vi "Package Measurement Plugin.vi"() -> ()   [LabVIEW 2021]
uses:
  _Measurement Plugin Packager/Packager Helpers/Queue Driver/controls/Queue Operations.ctl
  <vilib>/Utility/miscctls.llb/LVRowAndColumnTypeDef.ctl
  _Measurement Plugin Packager/Packager Helpers/controls/Config File Operations.ctl
  _Measurement Plugin Packager/Packager Helpers/controls/Data Holder.ctl
  <vilib>/Utility/miscctls.llb/LVPoint32TypeDef.ctl
  _Measurement Plugin Packager/Packager Helpers/controls/Build Spec Details.ctl
  <vilib>/AppBuilder/AB_API_Simple/Get Build Specification Version (path).vi
  _Measurement Plugin Packager/Packager Helpers/Queue Driver/Queue Driver.lvlib
  _Measurement Plugin Packager/Packager Helpers/Packager Helpers.lvlib
  _Measurement Plugin Packager/Packager Helpers/Dictionary/Dictionary.lvlib
  <vilib>/AppBuilder/AB_API_Simple/NI_App_Builder_API.lvlib
panel:
  out "error out":errorcluster
  out "Tab Control":T1(tab)
  in  "Open Directory":bool
  in  "Feed Path":path
  out "Warning":bool=TRUE caption="Existing LabVIEW Project Path should be selected"
  in  "Next to select":bool
  in  "Project":path caption="LabVIEW Project Path"
  in  "Feed":T2(radio)
  in  "Back 1":bool
  in  "Populate Package":bool
  in  "Select All":bool
  out "Measurement List":i32(listbox)=-1 caption="Select the Measurements to build the package"
  out "Selection warning":string="Selected Project doesn't have EXE build spec"
  out "Maintainer Warning":string
  in  "Settings Page":enum32{"Page 1", "Page 2"}(tab)
  in  "Maintainer Email ID":string="sabthagiri@ni.com"
  in  "Architecture":string(combo)="1"
  in  "Maintainer":string="NI"
  in  "Back 2":bool
  in  "Start Build":bool
  in  "Package List":i32[](listbox) caption="Edit the Package Name and Version"
  in  "Settings":bool
  in  "Progres Bar":i32(slide)=9 caption="Creating Distribution..." scale=0.0..100.0
  in  "Start Next":bool
  in  "Build Status":i32(listbox)=-1
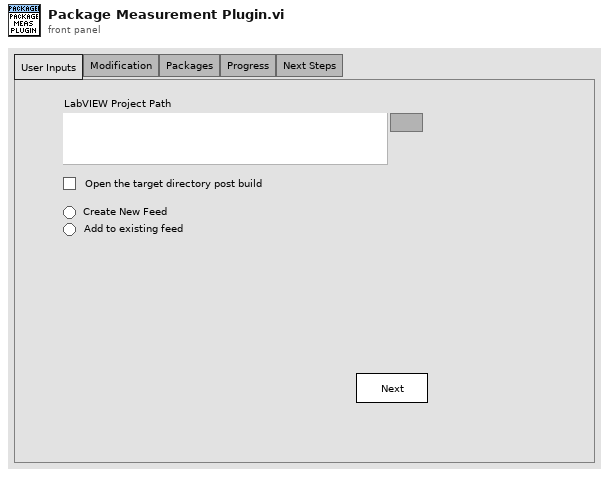
[diagram p1: front panel]
types:
  T1 = enum32{"User Inputs", "Modification", "Packages", "Progress", "Next Steps"}
  T2 = enum32{"No Selection", "CreateFeed", "AddtoFeed"}
  T3 = typedef "LVRowAndColumnTypeDef.ctl" = cluster{"Row":i32, "Column":i32}
  T4 = typedef "Queue Driver.lvlib/Queue Operations.ctl" = enum16{"Create Q", "Enqueue", "Enqueue N", "Dequeue", "Flush", "Release"}
  T5 = enum8{"Enabled", "Disabled", "Disabled and Grayed Out"}
  T6 = typedef "Packager Helpers.lvlib/Config File Operations.ctl" = enum16{"Read", "Write"}
  T7 = typedef "Packager Helpers.lvlib/Data Holder.ctl" = cluster{"Next Clicked?":bool, "MosueDown Coords":T8, "Build Spec":T9[], "No of Meas":i32, "No. of Selected Meas":i32, "Selected Meas":T9[], "Package Details":string[][], "Packages Path":path, "Feed":enum32{"No Selection", "CreateFeed", "AddtoFeed"}, "Feed Path":path, "Valid Inputs?":bool, "Feed Old":enum32{"No Selection", "CreateFeed", "AddtoFeed"}, "Status":string[], "Open Directory?":bool}
  T8 = typedef "LVPoint32TypeDef.ctl" = cluster{"Horizontal":i32, "Vertical":i32}
  T9 = typedef "Packager Helpers.lvlib/Build Spec Details.ctl" = cluster{"EXE Name":string, "Target path":path, "Has PPL?":bool, "PPL Name":string}
  T10 = typedef "NI_App_Builder_API.lvlib/Build Specification Version.ctl" = cluster{"Major":u16, "Minor":u16, "Fix":u16, "Build":u16}
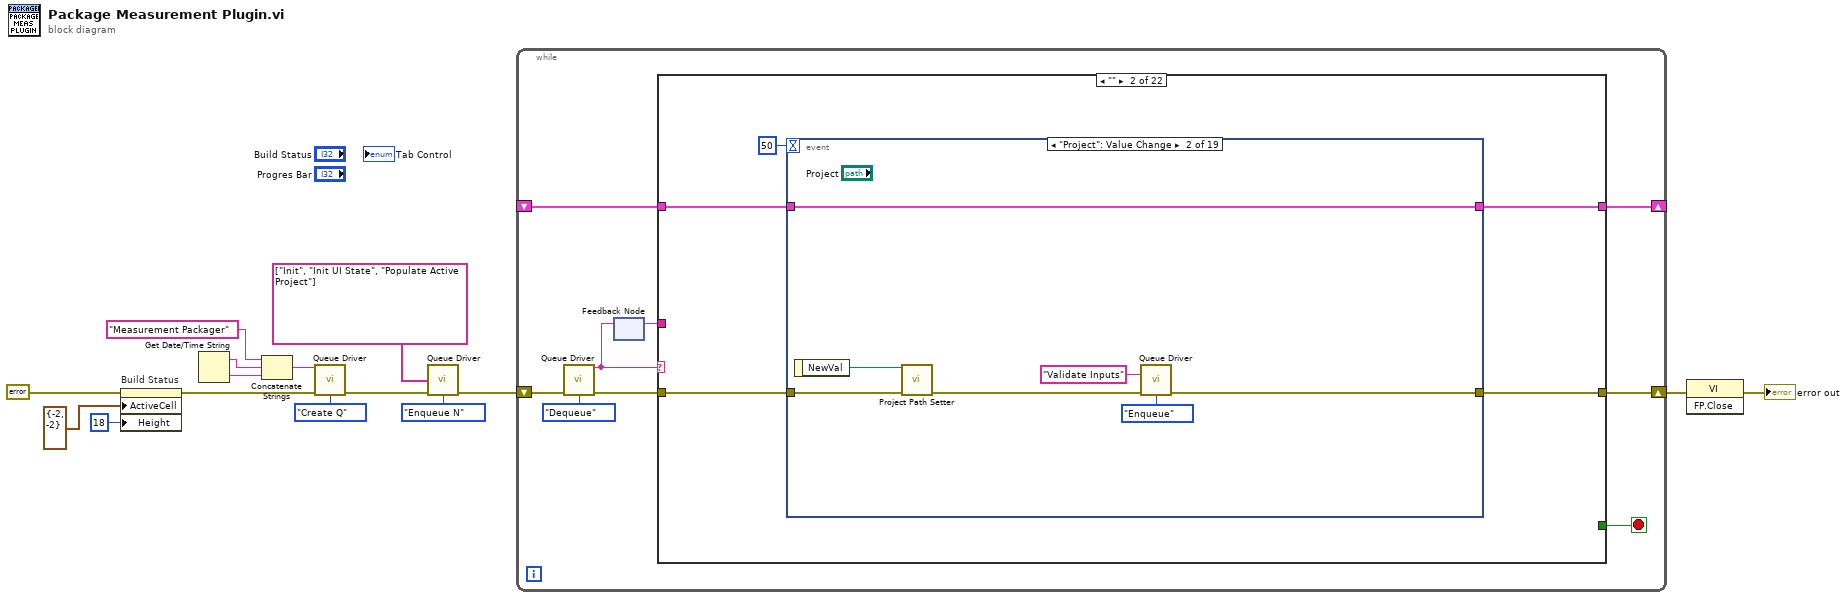
[diagram p0: block diagram]
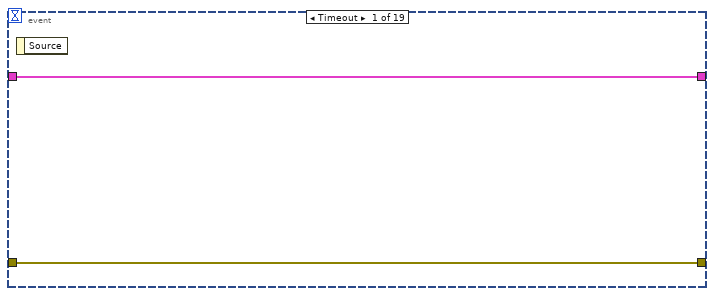
[diagram p3: hidden frame]
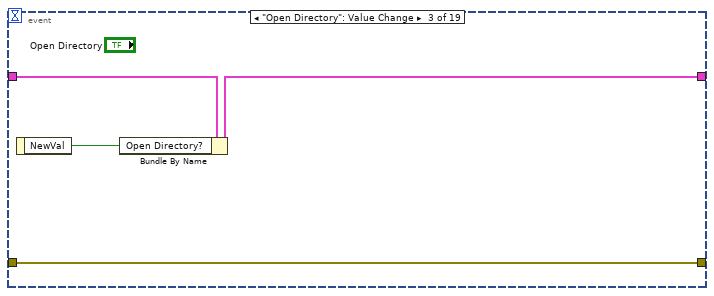
[diagram p4: hidden frame]
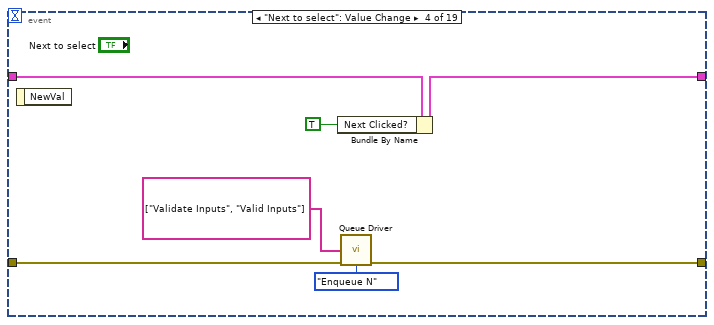
[diagram p5: hidden frame]
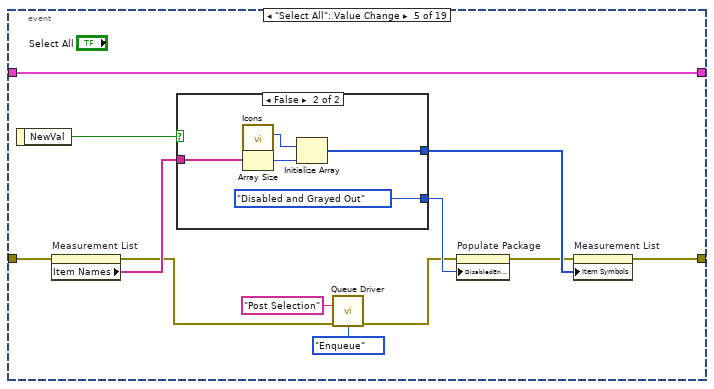
[diagram p6: hidden frame]
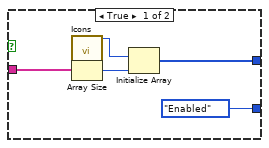
[diagram p7: hidden frame]
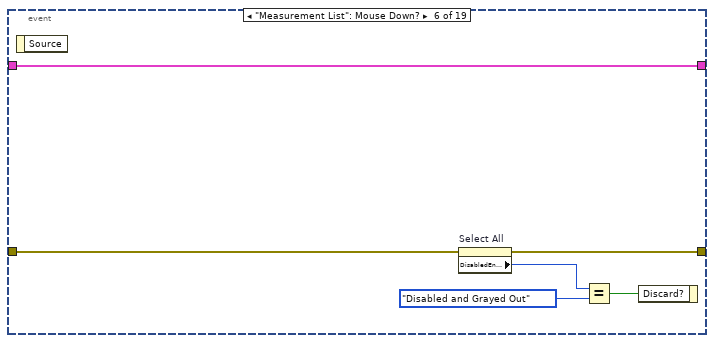
[diagram p8: hidden frame]
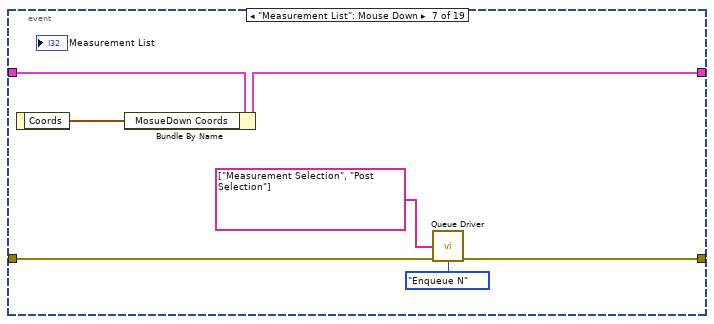
[diagram p9: hidden frame]
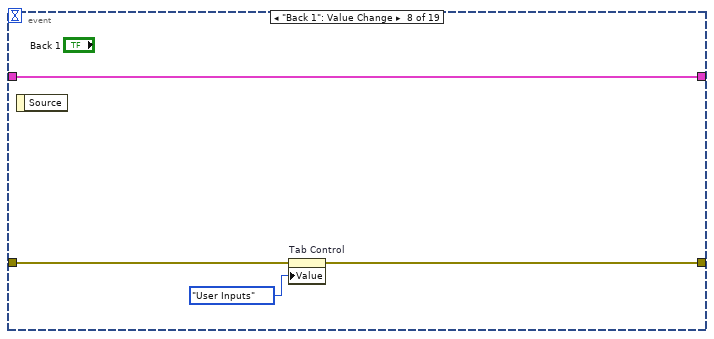
[diagram p10: hidden frame]
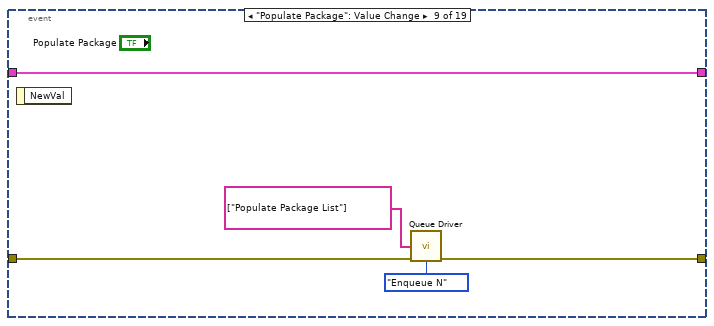
[diagram p11: hidden frame]
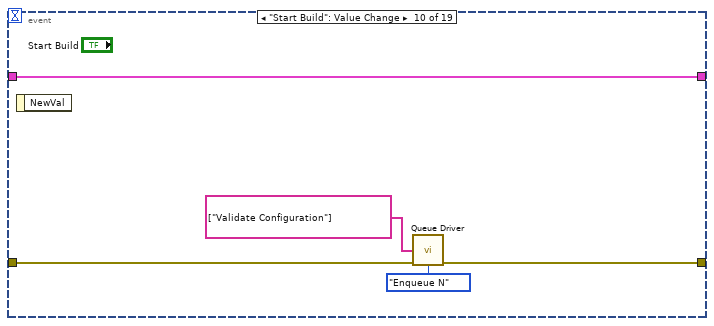
[diagram p12: hidden frame]
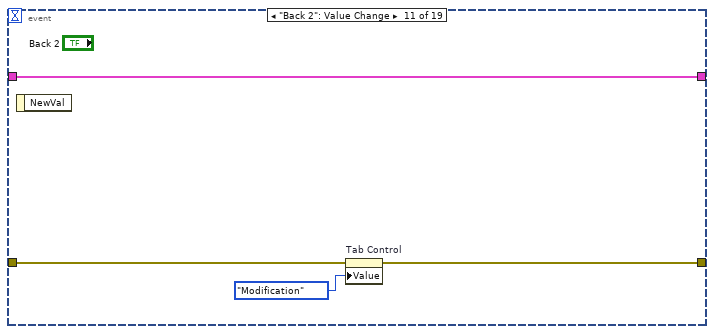
[diagram p13: hidden frame]
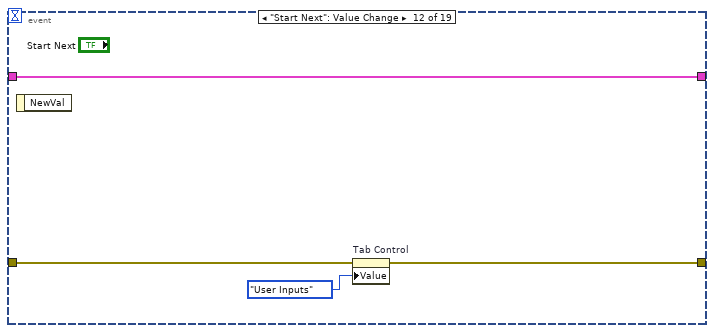
[diagram p14: hidden frame]
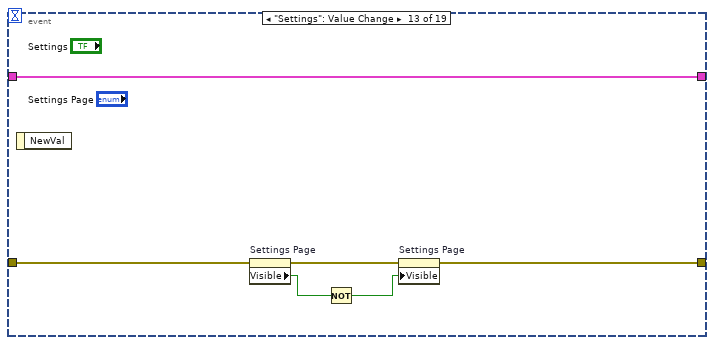
[diagram p15: hidden frame]
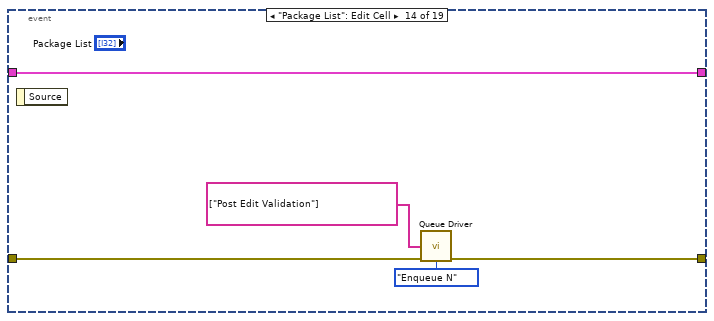
[diagram p16: hidden frame]
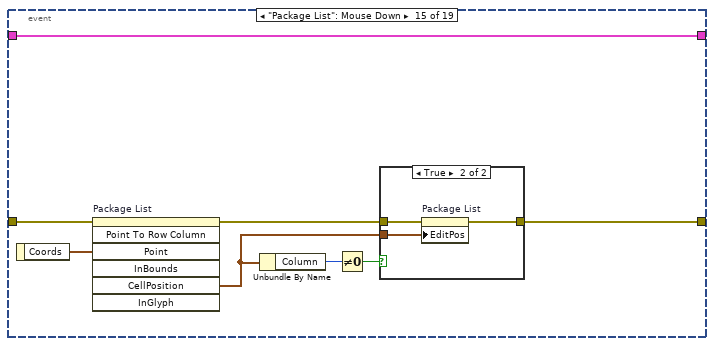
[diagram p17: hidden frame]
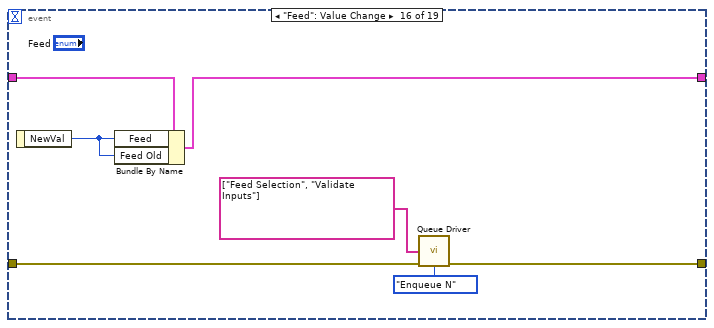
[diagram p19: hidden frame]
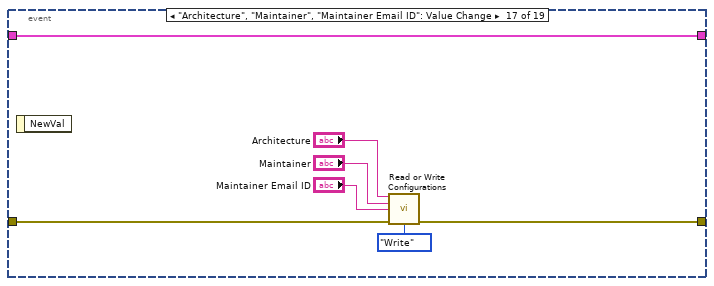
[diagram p20: hidden frame]
diagram:
  n1 = property on="Build Status" class="MCListbox (strict)"(error in=errorcluster {"status"=FALSE, "code"=0, "source"=""} ("error in (no error)"), "ActiveCell"=T3 {"Row"=-2, "Column"=-2} ("Active Cell:Active Cell"), "Height"=u32 18 ("Active Cell:Cell Size:Height")) -> (error out=w1:errorcluster)  [unwired: 1 in, 1 out]
  n2 = Get Date/Time String() -> (date string=w4:string, time string=w10:string)  [unwired: 3 in]
  n3 = Concatenate Strings("Measurement Packager" ("string"), w4, w10) -> (w9:string)
  n4 = call "Queue Driver.vi"("Name"=w9, "error in (no error)"=w1, "Queue Operations"=Queue_Operations."Create Q" ("Q Operations")) -> ("error out"=w13:errorcluster)  [unwired: 11 in, 1 out]
  n5 = call "Queue Driver.vi"("States[]"=string[] ["Init", "Init UI State", "Populate Active Project"], "error in (no error)"=w13, "Queue Operations"=Queue_Operations."Enqueue N" ("Q Operations")) -> ("error out"=w15:errorcluster)  [unwired: 11 in, 1 out]
  n6 = while {
    shift-right: [w17] -> w6
    shift-left: w15 -> [w24]
    shift-right: [w21] -> _
    shift-left: _ -> [w20]
    stop <- w18 stop-if-true
    n7 = call "Queue Driver.vi"("error in (no error)"=w24, "Queue Operations"=Queue_Operations."Dequeue" ("Q Operations")) -> ("Dequeued State"=w16:string, "error out"=w22:errorcluster)  [unwired: 12 in]
    n8 = feedback #1() -> (w19:string)  [unwired: 1 in]
    n9 = feedback-in #1(w16) -> ()
    n10 = case shown="\"\"" w16 {
      tunnel: w22 -> [w25 w31 w163 w176 w187 w190 w203 w243 w258 w273 w296 w315 w329 w336 w356 w392 w396 w410 w425 w439 w452 w457]
      tunnel: [w25 w27 w161 w167 w184 w189 w206 w242 w257 w270 w288 w316 w328 w333 w350 w391 w394 w407 w420 w437 w448 w459] -> w17
      tunnel: [w26 w30 w164 w179 w188 w191 w205 w241 w259 w275 w298 w323 w331 w342 w359 w393 w397 w403 w436 w441 w455 w460] -> w21
      tunnel: w20 -> [w26 w29 _ w179 w188 w191 w204 w241 w259 w275 w298 w324 w331 w342 w357 w393 w399 w403 w432 w441 w455 w460]
      tunnel: w19 -> [_ _ _ _ _ _ _ _ _ _ _ _ _ _ _ _ _ _ _ _ _ _]
      tunnel: [_ _ _ _ _ _ _ _ _ _ _ _ _ _ _ _ _ _ _ _ _ TRUE] -> w18
      frame Default {
      }
      frame "" {
        n11 = event shown="[1] \"Project\": Value Change" {
          selector: _ -> [_ _ _ _ _ _ _ _ _ _ _ _ _ _ _ _ _ _ _]
          dyn-events: _ -> [_ _ _ _ _ _ _ _ _ _ _ _ _ _ _ _ _ _ _]
          timeout: 50 -> [_ _ _ _ _ _ _ _ _ _ _ _ _ _ _ _ _ _ _]
          tunnel: [w32 w34 w41 w45 w52 w77 w81 w87 w93 w96 w103 w107 w111 w115 w121 w133 w139 w147 w153] -> w27
          tunnel: w31 -> [w32 w36 w41 w46 w56 w78 w80 w88 w94 w97 w104 w108 w112 w116 w120 w134 w140 w148 w154]
          tunnel: [w33 w39 w43 w49 w63 w79 w85 w90 w95 w100 w102 w106 w109 w119 w127 w137 w145 w151 w157] -> w30
          tunnel: w29 -> [w33 w39 w44 w50 w63 w79 w86 w90 w95 w100 w102 w106 w109 w119 w127 w138 w145 w152 w157]
          event Timeout {
            n12 = event-data() -> ()  [unwired: 1 in, 1 out]
          }
          event "Project": Value Change {
            n13 = event-data() -> ("NewVal"=w38:path)  [unwired: 1 in]
            n14 = call "Project Path Setter.vi"("ProjectPath In"=w38, "error in (no error)"=w36) -> ("error out"=w35:errorcluster)  [unwired: 13 in]
            n15 = call "Queue Driver.vi"("State"="Validate Inputs", "error in (no error)"=w35, "Queue Operations"=Queue_Operations."Enqueue" ("Q Operations")) -> ("error out"=w34:errorcluster)  [unwired: 11 in, 1 out]
          }
          event "Open Directory": Value Change {
            n16 = event-data() -> ("NewVal"=w42:bool)  [unwired: 1 in]
            n17 = Bundle By Name(cluster=w44, "Open Directory?"=w42) -> (w43:T7)
          }
          event "Next to select": Value Change {
            n18 = event-data() -> ()  [unwired: 1 in, 1 out]
            n19 = Bundle By Name(cluster=w50, "Next Clicked?"=TRUE) -> (w49:T7)
            n20 = call "Queue Driver.vi"("States[]"=string[] ["Validate Inputs", "Valid Inputs"], "error in (no error)"=w46, "Queue Operations"=Queue_Operations."Enqueue N" ("Q Operations")) -> ("error out"=w45:errorcluster)  [unwired: 11 in, 1 out]
          }
          event "Select All": Value Change {
            n21 = event-data() -> ("NewVal"=w58:bool)  [unwired: 1 in]
            n22 = property on="Measurement List" class="LstBox (strict)"(error in=w56) -> (error out=w55:errorcluster, "Item Names"=w62:string[])  [unwired: 1 in, 1 out]
            n23 = case shown="False" w58 {
              tunnel: w62 -> [w67 w72]
              tunnel: [w66 w71] -> w61
              tunnel: [T5."Enabled" ("Disabled") T5."Disabled and Grayed Out" ("Disabled")] -> w60
              frame True {
                n24 = call "Icons.vi"() -> ("Selected"=w64:i32)  [unwired: 14 in, 1 out]
                n25 = Array Size(array=w67) -> (size(s)=w68:i32)
                n26 = Initialize Array(w64, w68) -> (w66:i32[])
              }
              frame False {
                n27 = call "Icons.vi"() -> ("Non Selected"=w70:i32)  [unwired: 14 in, 1 out]
                n28 = Array Size(array=w72) -> (size(s)=w73:i32)
                n29 = Initialize Array(w70, w73) -> (w71:i32[])
              }
            }
            n30 = call "Queue Driver.vi"("State"="Post Selection", "error in (no error)"=w55, "Queue Operations"=Queue_Operations."Enqueue" ("Q Operations")) -> ("error out"=w54:errorcluster)  [unwired: 11 in, 1 out]
            n31 = property on="Populate Package" class="Bool"(error in=w54, "DisabledEnum"=w60) -> (error out=w53:errorcluster)  [unwired: 1 in, 1 out]
            n32 = property on="Measurement List" class="LstBox (strict)"(error in=w53, "Item Symbols"=w61) -> (error out=w52:errorcluster)  [unwired: 1 in, 1 out]
          }
          event "Measurement List": Mouse Down? {
            n33 = event-data() -> ()  [unwired: 1 in, 1 out]
            n34 = property on="Select All" class="Bool (strict)"(error in=w78) -> (error out=w77:errorcluster, "DisabledEnum"=w76:T5)  [unwired: 1 in, 1 out]
            n35 = Equal?(x=w76, y=T5."Disabled and Grayed Out") -> (x = y?=w74:bool)
            n36 = event-data("Discard?"=w74) -> ()  [unwired: 1 in, 1 out]
          }
          event "Measurement List": Mouse Down {
            n37 = event-data() -> ("Coords"=w83:T8)  [unwired: 1 in]
            n38 = Bundle By Name(cluster=w86, "MosueDown Coords"=w83) -> (w85:T7)
            n39 = call "Queue Driver.vi"("States[]"=string[] ["Measurement Selection", "Post Selection"], "error in (no error)"=w80, "Queue Operations"=Queue_Operations."Enqueue N" ("Q Operations")) -> ("error out"=w81:errorcluster)  [unwired: 11 in, 1 out]
          }
          event "Back 1": Value Change {
            n40 = event-data() -> ()  [unwired: 1 in, 1 out]
            n41 = property on="Tab Control" class="TabCtl (strict)"(error in=w88, "Value"=T1."User Inputs" ("Tab Control")) -> (error out=w87:errorcluster)  [unwired: 1 in, 1 out]
          }
          event "Populate Package": Value Change {
            n42 = event-data() -> ()  [unwired: 1 in, 1 out]
            n43 = call "Queue Driver.vi"("States[]"=string[] ["Populate Package List"], "error in (no error)"=w94, "Queue Operations"=Queue_Operations."Enqueue N" ("Q Operations")) -> ("error out"=w93:errorcluster)  [unwired: 11 in, 1 out]
          }
          event "Start Build": Value Change {
            n44 = event-data() -> ()  [unwired: 1 in, 1 out]
            n45 = call "Queue Driver.vi"("States[]"=string[] ["Validate Configuration"], "error in (no error)"=w97, "Queue Operations"=Queue_Operations."Enqueue N" ("Q Operations")) -> ("error out"=w96:errorcluster)  [unwired: 11 in, 1 out]
          }
          event "Back 2": Value Change {
            n46 = event-data() -> ()  [unwired: 1 in, 1 out]
            n47 = property on="Tab Control" class="TabCtl (strict)"(error in=w104, "Value"=T1."Modification" ("Tab Control")) -> (error out=w103:errorcluster)  [unwired: 1 in, 1 out]
          }
          event "Start Next": Value Change {
            n48 = event-data() -> ()  [unwired: 1 in, 1 out]
            n49 = property on="Tab Control" class="TabCtl (strict)"(error in=w108, "Value"=T1."User Inputs" ("Tab Control")) -> (error out=w107:errorcluster)  [unwired: 1 in, 1 out]
          }
          event "Settings": Value Change {
            n50 = event-data() -> ()  [unwired: 1 in, 1 out]
            n51 = property on="Settings Page" class="TabCtl (strict)"(error in=w112) -> (error out=w110:errorcluster, "Visible"=w114:bool)  [unwired: 1 in, 1 out]
            n52 = Not(x=w114) -> (.not. x?=w113:bool)
            n53 = property on="Settings Page" class="TabCtl (strict)"(error in=w110, "Visible"=w113) -> (error out=w111:errorcluster)  [unwired: 1 in, 1 out]
          }
          event "Package List": Edit Cell {
            n54 = event-data() -> ()  [unwired: 1 in, 1 out]
            n55 = call "Queue Driver.vi"("States[]"=string[] ["Post Edit Validation"], "error in (no error)"=w116, "Queue Operations"=Queue_Operations."Enqueue N" ("Q Operations")) -> ("error out"=w115:errorcluster)  [unwired: 11 in, 1 out]
          }
          event "Package List": Mouse Down {
            n56 = event-data() -> ("Coords"=w126:T8)  [unwired: 1 in]
            n57 = invoke on="Package List" class="MCListbox (strict)" method="Point To Row Column"(error in=w120, "Point"=w126) -> (error out=w122:errorcluster, "CellPosition"=w123:T3)  [unwired: 5 in, 5 out]
            n58 = Unbundle By Name(w123) -> ("Column"=w125:i32)
            n59 = Not Equal To 0?(x=w125) -> (x != 0?=w124:bool)
            n60 = case shown="True" w124 {
              tunnel: w123 -> [_ w131]
              tunnel: w122 -> [w128 w130]
              tunnel: [w128 w129] -> w121
              frame False {
              }
              frame True {
                n61 = property on="Package List" class="MCListbox (strict)"(error in=w130, "EditPos"=w131) -> (error out=w129:errorcluster)  [unwired: 1 in, 1 out]
              }
            }
          }
          event "Feed": Value Change {
            n62 = event-data() -> ("NewVal"=w132:T2)  [unwired: 1 in]
            n63 = Bundle By Name(cluster=w138, "Feed"=w132, "Feed Old"=w132) -> (w137:T7)
            n64 = call "Queue Driver.vi"("States[]"=string[] ["Feed Selection", "Validate Inputs"], "error in (no error)"=w134, "Queue Operations"=Queue_Operations."Enqueue N" ("Q Operations")) -> ("error out"=w133:errorcluster)  [unwired: 11 in, 1 out]
          }
          event "Architecture", "Maintainer", "Maintainer Email ID": Value Change {
            n65 = event-data() -> ()  [unwired: 1 in, 1 out]
            n66 = call "Read or Write Configurations.vi"("Architecture"="Architecture", "Maintainer"="Maintainer", "Email"="Maintainer Email ID", "error in (no error)"=w140, "Operation"=Config_File_Operations."Write") -> ("error out"=w139:errorcluster)  [unwired: 7 in, 3 out]
          }
          event "Feed Path": Value Change {
            n67 = event-data() -> ("NewVal"=w149:path)  [unwired: 1 in]
            n68 = Bundle By Name(cluster=w152, "Feed Path"=w149) -> (w151:T7)
            n69 = call "Queue Driver.vi"("States[]"=string[] ["Validate Inputs"], "error in (no error)"=w148, "Queue Operations"=Queue_Operations."Enqueue N" ("Q Operations")) -> ("error out"=w147:errorcluster)  [unwired: 11 in, 1 out]
          }
          event Panel Close? {
            n70 = event-data() -> ()  [unwired: 1 in, 4 out]
            n71 = call "Queue Driver.vi"("State"="Exit", "error in (no error)"=w154, "Queue Operations"=Queue_Operations."Enqueue" ("Q Operations")) -> ("error out"=w153:errorcluster)  [unwired: 11 in, 1 out]
            n72 = event-data("Discard?"=TRUE) -> ()  [unwired: 1 in, 1 out]
          }
        }
      }
      frame "Init" {
        w160 = TRUE ("Open Directory?")
        w159 = T2."No Selection" ("Feed")
        n73 = invoke class="VI" method="Default Vals.Reinit All"(error in=w163) -> (error out=w162:errorcluster)  [unwired: 2 in, 2 out]
        n74 = property on="Open Directory" class="Bool (strict)"(error in=w162, "Value"=w160) -> (error out=w161:errorcluster)  [unwired: 1 in, 1 out]
        n75 = Bundle By Name(cluster=T7 {"Next Clicked?"=TRUE, "MosueDown Coords"={"Horizontal"=0, "Vertical"=0}, "Build Spec"=[], "No of Meas"=0, "No. of Selected Meas"=0, "Selected Meas"=[], "Package Details"=[], "Packages Path"=path "", "Feed"=enum."No Selection", "Feed Path"=path "", "Valid Inputs?"=FALSE, "Feed Old"=enum."No Selection", "Status"=[], "Open Directory?"=FALSE}, "Feed"=w159, "Feed Old"=w159, "Open Directory?"=w160) -> (w164:T7)
      }
      frame "Init UI State" {
        w177 = u32 16448250 ("Selection Color")
        w166 = FALSE ("Visible")
        n76 = property on="Tab Control" class="TabCtl (strict)"(error in=w176, "Value"=T1."User Inputs" ("Tab Control")) -> (error out=w175:errorcluster)  [unwired: 1 in, 1 out]
        n77 = property on="Settings Page" class="TabCtl (strict)"(error in=w175, "Visible"=w166) -> (error out=w174:errorcluster)  [unwired: 1 in, 1 out]
        n78 = property on="Warning" class="Bool"(error in=w174, "Visible"=w166) -> (error out=w173:errorcluster)  [unwired: 1 in, 1 out]
        n79 = property on="Selection warning" class="Str"(error in=w173, "Visible"=w166) -> (error out=w172:errorcluster)  [unwired: 1 in, 1 out]
        n80 = property on="Feed Path" class="Path"(error in=w172, "Visible"=w166) -> (error out=w171:errorcluster)  [unwired: 1 in, 1 out]
        n81 = property on="Settings" class="Bool"(error in=w171, "Visible"=w166) -> (error out=w170:errorcluster)  [unwired: 1 in, 1 out]
        n82 = property on="Measurement List" class="LstBox (strict)"(error in=w170, "SelColor"=w177) -> (error out=w169:errorcluster)  [unwired: 1 in, 1 out]
        n83 = property on="Package List" class="MCListbox (strict)"(error in=w169, "SelColor"=w177) -> (error out=w168:errorcluster)  [unwired: 1 in, 1 out]
        n84 = property on="Build Status" class="MCListbox (strict)"(error in=w168, "SelColor"=w177) -> (error out=w167:errorcluster)  [unwired: 1 in, 1 out]
        "Selection warning" <- "Atleast one measurement should be selected" ("Selection warning")
        "Maintainer Warning" <- "Maintainer and Email ID cannot be empty" ("Maintainer Warning")
        "Warning" <- TRUE ("Warning")
      }
      frame "Populate Active Project" {
        # "Get the active labview project"
        n85 = call "Get Active ProjectPath.vi"("error in (no error)"=w187) -> ("Project Path"=w183:path, "error out"=w186:errorcluster)  [unwired: 13 in]
        n86 = property on="Project" class="Path"(error in=w186, "Value"=w183) -> (error out=w185:errorcluster)  [unwired: 1 in, 1 out]
        n87 = call "Project Path Setter.vi"("ProjectPath In"=w183, "error in (no error)"=w185) -> ("error out"=w184:errorcluster)  [unwired: 13 in]
      }
      frame "Populate Config" {
        # "Disabling it because the config will not be populated in UI"
        # "Populate Config Data"
        n88 = disable-structure shown="Enabled" {
          disable-tunnel: w190 -> [w196 w201]
          disable-tunnel: [w192 w201] -> w189
          frame Disabled {
            n89 = call "Read or Write Configurations.vi"("error in (no error)"=w196, "Operation"=Config_File_Operations."Read") -> ("Architecture Out"=w199:string, "Maintainer Out"=w198:string, "Email Out"=w197:string, "error out"=w195:errorcluster)  [unwired: 10 in]
            n90 = property on="Maintainer Email ID" class="Str"(error in=w195, "Value"=w197) -> (error out=w194:errorcluster)  [unwired: 1 in, 1 out]
            n91 = property on="Maintainer" class="Str"(error in=w194, "Value"=w198) -> (error out=w193:errorcluster)  [unwired: 1 in, 1 out]
            n92 = property on="Architecture" class="CmbBox"(error in=w193, "Value"=w199) -> (error out=w192:errorcluster)  [unwired: 1 in, 1 out]
          }
          frame Enabled {
          }
        }
      }
      frame "Validate Inputs" {
        # "Validate Inputs"
        n93 = call "Validate Project Path.vi"("error in (no error)"=w203) -> ("Valid Path?"=w202:bool, "error out"=w207:errorcluster)  [unwired: 13 in]
        n94 = case "Valid project?" shown="True" w202 {
          tunnel: w207 -> [w214 w215]
          tunnel: [w213 w216] -> w206
          tunnel: [w211 w217] -> w205
          tunnel: w204 -> [w212 w218]
          frame False {
            # "Invalid project Path"
            n95 = Bundle By Name(cluster=w212, "Valid Inputs?"=FALSE) -> (w211:T7)
            n96 = property on="Warning" class="Bool"(error in=w214, "Visible"=TRUE, "Caption.Text"="Existing LabVIEW Project Path should be selected" ("Boolean Text.Text")) -> (error out=w213:errorcluster)  [unwired: 1 in, 1 out]
          }
          frame True {
            n97 = Unbundle By Name(w218) -> ("Feed"=w220:T2, "Feed Path"=w219:path)
            n98 = case shown="\"AddtoFeed\"" w220 {
              tunnel: w215 -> [w228 w234]
              tunnel: w219 -> [w229 _]
              tunnel: w218 -> [w233 w239]
              tunnel: [w232 w238] -> w217
              tunnel: [w231 w235] -> w216
              frame "AddtoFeed" {
                # "Validate Path"
                n99 = Empty String/Path?(string/path=w229) -> (empty?=w227:bool)
                n100 = Not A Number/Path/Refnum?(number/path/refnum=w229) -> (NaN/Path/Refnum?=w226:bool)
                n101 = call <vilib>:"Check if File or Folder Exists.vi"("error in (no error)"=w228, "path"=w229) -> ("error out"=w224:errorcluster, "file or folder exists?"=w225:bool)  [unwired: 7 in, 1 out]
                n102 = Not(x=w225) -> (.not. x?=w223:bool)
                n103 = Compound Arithmetic op=OR(w227, w226, w223) -> (w222:bool)
                n104 = Not(x=w222) -> (.not. x?=w230:bool)
                n105 = Bundle By Name(cluster=w233, "Valid Inputs?"=w230) -> (w232:T7)
                n106 = property on="Warning" class="Bool"(error in=w224, "Visible"=w222, "Caption.Text"="Feed Path cannot be empty/invalid" ("Boolean Text.Text")) -> (error out=w231:errorcluster)  [unwired: 1 in, 1 out]
              }
              frame Default {
                n107 = property on="Warning" class="Bool"(error in=w234, "Visible"=FALSE) -> (error out=w235:errorcluster)  [unwired: 1 in, 1 out]
                n108 = Bundle By Name(cluster=w239, "Valid Inputs?"=TRUE) -> (w238:T7)
              }
            }
          }
        }
      }
      frame "Valid Inputs" {
        # "Check if valid inputs and if next is clicked"
        n109 = Unbundle By Name(w241) -> ("Valid Inputs?"=w240:bool)
        n110 = case "Valid Inputs?" shown="True" w240 {
          tunnel: w243 -> [w244 w250]
          tunnel: [w244 w247] -> w242
          tunnel: w241 -> [_ w246]
          frame False {
          }
          frame True {
            n111 = Unbundle By Name(w246) -> ("Next Clicked?"=w245:bool)
            n112 = property on="Warning" class="Bool"(error in=w250, "Visible"=FALSE) -> (error out=w248:errorcluster)  [unwired: 1 in, 1 out]
            n113 = case "Next Clicked?" shown="True" w245 {
              tunnel: w248 -> [w251 w254]
              tunnel: [w251 w252] -> w247
              frame False {
              }
              frame True {
                n114 = call "Queue Driver.vi"("States[]"=string[] ["Populate Measurements", "Update Tab", "Validate Measurement"], "error in (no error)"=w254, "Queue Operations"=Queue_Operations."Enqueue N" ("Q Operations")) -> ("error out"=w252:errorcluster)  [unwired: 11 in, 1 out]
              }
            }
          }
        }
      }
      frame "Feed Selection" {
        # "Feed Selection Value Change Handling"
        n115 = Unbundle By Name(w259) -> ("Feed"=w256:T2)
        n116 = case shown="Default" w256 {
          tunnel: w258 -> [w262 w265]
          tunnel: [w261 w264] -> w257
          frame Default {
            n117 = property on="Feed Path" class="Path"(error in=w262, "Visible"=FALSE) -> (error out=w261:errorcluster)  [unwired: 1 in, 1 out]
          }
          frame "AddtoFeed" {
            n118 = property on="Feed Path" class="Path"(error in=w265, "Visible"=TRUE) -> (error out=w264:errorcluster)  [unwired: 1 in, 1 out]
          }
        }
      }
      frame "Measurement Selection" {
        # "Measurement Selection Value change"
        n119 = Unbundle By Name(w275) -> ("No of Meas"=w267:i32, "MosueDown Coords"=w266:T8)
        n120 = property on="Measurement List" class="LstBox (strict)"(error in=w273) -> (error out=w272:errorcluster, "Item Symbols"=w274:i32[])  [unwired: 1 in, 1 out]
        n121 = invoke on="Measurement List" class="LstBox (strict)" method="Point To Row"(error in=w272, "Point"=w266) -> (error out=w271:errorcluster, "Row"=w269:i32)  [unwired: 5 in, 5 out]
        n122 = Greater?(x=w267, y=w269) -> (0:w268:bool)
        n123 = case "Mouse click In range?" shown="True" w268 {
          tunnel: w274 -> [_ w281]
          tunnel: w269 -> [_ w277]
          tunnel: w271 -> [w276 w279]
          tunnel: [w276 w278] -> w270
          frame False {
          }
          frame True {
            # "Change the item symbols"
            n124 = in-place {
              n125 = in-place-array #2(w281, w277) -> (w285:i32)
              n126 = call "Icons.vi"() -> ("Selected"=w282:i32, "Non Selected"=w286:i32)  [unwired: 14 in]
              n127 = Equal?(x=w285, y=w282) -> (x = y?=w284:bool)
              n128 = Swap Values(12:w282, 13:w284, 14:w286) -> (1:w283:i32)  [unwired: 1 out]
              n129 = in-place-array #2(w283) -> (w280:i32[])  [unwired: 1 out]
            }
            n130 = property on="Measurement List" class="LstBox (strict)"(error in=w279, "Item Symbols"=w280) -> (error out=w278:errorcluster)  [unwired: 1 in, 1 out]
          }
        }
      }
      frame "Post Selection" {
        # "Selection change handling"
        n131 = property on="Measurement List" class="LstBox (strict)"(error in=w296) -> (error out=w295:errorcluster, "Item Symbols"=w297:i32[])  [unwired: 1 in, 1 out]
        n132 = call "Check the Symbols.vi"("Item Symbols"=w297) -> ("All Selected?"=w287:bool, "None Selected"=w292:bool)  [unwired: 13 in]
        n133 = case "All selected?" shown="False" w287 {
          tunnel: [w304 T5."Enabled" ("Disabled")] -> w291
          tunnel: w295 -> [w301 w314]
          tunnel: [w303 w312] -> w294
          tunnel: w292 -> [w302 _]
          tunnel: [w299 _] -> w290
          frame False {
            n134 = property on="Select All" class="Bool (strict)"(error in=w301, "Value"=FALSE ("All")) -> (error out=w300:errorcluster)  [unwired: 1 in, 1 out]
            n135 = case "None Selected?" shown="False" w302 {
              tunnel: [T5."Enabled" ("Disabled") T5."Disabled and Grayed Out" ("Disabled")] -> w304
              tunnel: [w306 w309] -> w303
              tunnel: w300 -> [w306 w309]
              tunnel: [_ TRUE] -> w299
              frame False {
              }
              frame True {
              }
            }
          }
          frame True {
            n136 = property on="Select All" class="Bool (strict)"(error in=w314, "Value"=TRUE ("All")) -> (error out=w312:errorcluster)  [unwired: 1 in, 1 out]
          }
        }
        n137 = property on="Populate Package" class="Bool"(error in=w294, "DisabledEnum"=w291) -> (error out=w293:errorcluster)  [unwired: 1 in, 1 out]
        n138 = property on="Selection warning" class="Str"(error in=w293, "Visible"=w290, "Value"="Atleast one measurement should be selected" ("Selection warning")) -> (error out=w288:errorcluster)  [unwired: 1 in, 1 out]
      }
      frame "Populate Measurements" {
        # "Populate the selected measurements with the package name"
        n139 = call "Get all Build Spec Details.vi"("error in (no error)"=w315) -> ("Build Spec Details"=w322:T9[], "error out"=w317:errorcluster)  [unwired: 13 in]
        n140 = for {
          tunnel: w322 -> [w327] mode=indexing
          tunnel: [w326] -> w320 mode=indexing
          tunnel: [w325] -> w319 mode=indexing
          n141 = Unbundle By Name(w327) -> ("EXE Name"=w326:string)
          n142 = call "Icons.vi"() -> ("Selected"=w325:i32)  [unwired: 14 in, 1 out]
        }
        n143 = Array Size(array=w320) -> (size(s)=w318:i32)
        n144 = Bundle By Name(cluster=w324, "Build Spec"=w322, "No of Meas"=w318, "No. of Selected Meas"=w318) -> (w323:T7)
        n145 = property on="Measurement List" class="LstBox (strict)"(error in=w317, "Item Names"=w320, "Item Symbols"=w319, "Active Row"=-1 ("Selection Mode")) -> (error out=w316:errorcluster)  [unwired: 1 in, 1 out]
      }
      frame "Update Tab" {
        n146 = property on="Tab Control" class="TabCtl (strict)"(error in=w329, "Value"=T1."Modification" ("Tab Control")) -> (error out=w328:errorcluster)  [unwired: 1 in, 1 out]
      }
      frame "Validate Measurement" {
        # "Validate measurements"
        n147 = Unbundle By Name(w342) -> ("Build Spec"=w338:T9[])
        n148 = Empty Array?(array=w338) -> (empty?=w337:bool)
        n149 = case shown="True" w337 {
          tunnel: [T5."Enabled" ("Disabled") T5."Disabled and Grayed Out" ("Disabled")] -> w341
          tunnel: [TRUE ("All") FALSE ("All")] -> w332
          frame False {
          }
          frame True {
          }
        }
        n150 = property on="Populate Package" class="Bool"(error in=w336, "DisabledEnum"=w341) -> (error out=w335:errorcluster)  [unwired: 1 in, 1 out]
        n151 = property on="Select All" class="Bool (strict)"(error in=w335, "Value"=w332, "DisabledEnum"=w341) -> (error out=w334:errorcluster)  [unwired: 1 in, 1 out]
        n152 = Not(x=w332) -> (.not. x?=w339:bool)
        n153 = property on="Selection warning" class="Str"(error in=w334, "Visible"=w339, "Value"="Selected Project doesn't have EXE build spec" ("Selection warning")) -> (error out=w333:errorcluster)  [unwired: 1 in, 1 out]
      }
      frame "Populate Package List" {
        # "Populate Package List"
        n154 = property on="Measurement List" class="LstBox (strict)"(error in=w356) -> (error out=w355:errorcluster, "Item Names"=w363:string[], "Item Symbols"=w362:i32[])  [unwired: 1 in, 1 out]
        n155 = call "Project Path Getter.vi"("error in (no error)"=w355) -> ("Path"=w347:path, "error out"=w354:errorcluster)  [unwired: 13 in]
        n156 = for {
          tunnel: w363 -> [w369] mode=indexing
          tunnel: w362 -> [w371] mode=indexing
          tunnel: [w369] -> w361 mode=indexing if=w368
          tunnel: [w370] -> w358 mode=indexing if=w368
          shift-right: [w365] -> w353
          shift-left: w354 -> [w366]
          tunnel: w347 -> [w364]
          n157 = call "Icons.vi"() -> ("Selected"=w367:i32)  [unwired: 14 in, 1 out]
          n158 = Equal?(x=w371, y=w367) -> (x = y?=w368:bool)
          n159 = case shown="True" w368 {
            tunnel: [_ w384] -> w370
            tunnel: w366 -> [w372 w376]
            tunnel: w369 -> [_ w385]
            tunnel: [w372 w374] -> w365
            tunnel: w364 -> [_ w373]
            frame False {
            }
            frame True {
              n160 = call-poly <vilib>:"Get Build Specification Version.vi"("error in (no error)"=w376, "Name of build specification"=w385, "Path to project"=w373) -> ("error out"=w375:errorcluster, "Build Specification Version"=w379:T10)  [unwired: 7 in]
              n161 = call "Check Initial Version.vi"("Build Version In"=w379) -> ("Build Version Out"=w378:T10)  [unwired: 14 in]
              n162 = Unbundle By Name(w378) -> ("Major"=w383:u16, "Minor"=w382:u16, "Fix"=w381:u16, "Build"=w380:u16)
              n163 = Format Into String(format string="%d.%d.%d.%d", error in=w375, w383, w382, w381, w380) -> (resulting string=w384:string, error out=w374:errorcluster)  [unwired: 1 in]
            }
          }
        }
        n164 = Build Array(w361, w358) -> (w349:string[][])
        n165 = Transpose 2D Array(2D array=w349) -> (transposed array=w352:string[][])
        n166 = property on="Package List" class="MCListbox (strict)"(error in=w353, "ItemNames"=w352, "SelMode"=0 ("Selection Mode")) -> (error out=w351:errorcluster)  [unwired: 1 in, 1 out]
        n167 = Bundle By Name(cluster=w357, "Package Details"=w352) -> (w359:T7)
        n168 = property on="Tab Control" class="TabCtl (strict)"(error in=w351, "Value"=T1."Packages" ("Tab Control")) -> (error out=w350:errorcluster)  [unwired: 1 in, 1 out]
      }
      frame "Validate Configuration" {
        w389 = FALSE ("Visible")
        # "Check if configuration maintainer, maintainer email ID is valid"
        n169 = call "Queue Driver.vi"("States[]"=string[] ["Filter the Selected Measurements", "Build", "Post Build"], "error in (no error)"=w392, "Queue Operations"=Queue_Operations."Enqueue N" ("Q Operations")) -> ("error out"=w390:errorcluster)  [unwired: 11 in, 1 out]
        n170 = property on="Settings Page" class="TabCtl (strict)"(error in=w390, "Visible"=w389) -> (error out=w388:errorcluster)  [unwired: 1 in, 1 out]
        n171 = property on="Maintainer Warning" class="Str"(error in=w388, "Visible"=w389) -> (error out=w391:errorcluster)  [unwired: 1 in, 1 out]
      }
      frame "Filter the Selected Measurements" {
        # "Get the selected measurements"
        n172 = property on="Measurement List" class="LstBox (strict)"(error in=w396) -> (error out=w395:errorcluster, "Item Names"=w401:string[], "Item Symbols"=w402:i32[])  [unwired: 1 in, 1 out]
        n173 = Unbundle By Name(w399) -> ("Build Spec"=w400:T9[])
        n174 = call "Get Selected Measurements Data.vi"("Build Spec Details"=w400, "Item Names"=w401, "Item Symbols"=w402, "error in (no error)"=w395) -> ("Selected Measurements"=w398:T9[], "error out"=w394:errorcluster)  [unwired: 10 in]
        n175 = Bundle By Name(cluster=w399, "Selected Meas"=w398) -> (w397:T7)
      }
      frame "Post Edit Validation" {
        # "After editing validate if the changes are valid"
        n176 = Unbundle By Name(w403) -> ("Package Details"=w418:string[][])
        n177 = property on="Package List" class="MCListbox (strict)"(error in=w410) -> (error out=w409:errorcluster, "ItemNames"=w405:string[][])  [unwired: 1 in, 1 out]
        n178 = Index Array(array=w405, index (col)=1 ("disabled index (col)")) -> (element=w411:string[])  [unwired: 1 in]
        n179 = Index Array(array=w418, index (col) #1=0 ("disabled index (col)"), index (col) #2=1 ("disabled index (col)")) -> (element #1=w415:string[], element #2=w412:string[])  [unwired: 2 in]
        n180 = call "Validate the Version.vi"("Old Version"=w412, "New Version"=w411, "error in (no error)"=w409) -> ("Version Out"=w413:string[], "error out"=w408:errorcluster)  [unwired: 11 in]
        n181 = Build Array(w415, w413) -> (w414:string[][])
        n182 = Transpose 2D Array(2D array=w414) -> (transposed array=w406:string[][])
        n183 = property on="Package List" class="MCListbox (strict)"(error in=w408, "ItemNames"=w406) -> (error out=w407:errorcluster)  [unwired: 1 in, 1 out]
      }
      frame "Build" {
        # "Start build process"
        n184 = property on="Tab Control" class="TabCtl (strict)"(error in=w425, "Value"=T1."Progress" ("Tab Control")) -> (error out=w424:errorcluster)  [unwired: 1 in, 1 out]
        n185 = property on="Progres Bar" class="Slide (strict)"(error in=w424, "Value"=2 ("Progres Bar")) -> (error out=w423:errorcluster)  [unwired: 1 in, 1 out]
        n186 = Unbundle By Name(w432) -> ("Open Directory?"=w429:bool, "Feed"=w428:T2, "Feed Path"=w427:path, "Selected Meas"=w426:T9[])
        n187 = property on="Package List" class="MCListbox (strict)"(error in=w423) -> (error out=w422:errorcluster, "ItemNames"=w431:string[][])  [unwired: 1 in, 1 out]
        n188 = control-ref of="Progres Bar"() -> (w419:refnum<vi>)
        n189 = call "Start Build.vi"("Open Directory?"=w429, "Progres Bar"=w419, "Feed"=w428, "Feed Path"=w427, "Selected Measurements"=w426, "error in (no error)"=w422, "Package Spec"=w431) -> ("Status"=w430:string[], "error out"=w421:errorcluster)  [unwired: 7 in]
        n190 = Bundle By Name(cluster=w432, "Status"=w430) -> (w436:T7)
        n191 = property on="Tab Control" class="TabCtl (strict)"(error in=w421, "Value"=T1."Next Steps" ("Tab Control")) -> (error out=w420:errorcluster)  [unwired: 1 in, 1 out]
      }
      frame "Post Build" {
        # "Populate the results in post build"
        n192 = Unbundle By Name(w441) -> ("Selected Meas"=w440:T9[], "Status"=w443:string[])
        n193 = for {
          tunnel: w440 -> [w446] mode=indexing
          tunnel: [w445] -> w444 mode=indexing
          n194 = Unbundle By Name(w446) -> ("EXE Name"=w445:string)
        }
        n195 = Build Array(w444, w443) -> (w442:string[][])
        n196 = Transpose 2D Array(2D array=w442) -> (transposed array=w438:string[][])
        n197 = property on="Build Status" class="MCListbox (strict)"(error in=w439, "ItemNames"=w438) -> (error out=w437:errorcluster)  [unwired: 1 in, 1 out]
      }
      frame "Error" {
        n198 = call <vilib>:"Simple Error Handler.vi"("error in (no error)"=w452) -> ("error out"=w451:errorcluster)  [unwired: 4 in, 4 out]
        n199 = call <vilib>:"Clear Errors.vi"("error in (no error)"=w451) -> ("error out"=w450:errorcluster)  [unwired: 5 in, 1 out]
        n200 = call "Queue Driver.vi"("error in (no error)"=w450, "Queue Operations"=Queue_Operations."Flush" ("Q Operations")) -> ("error out"=w449:errorcluster)  [unwired: 12 in, 1 out]
        n201 = call "Queue Driver.vi"("State"="Exit", "error in (no error)"=w449, "Queue Operations"=Queue_Operations."Enqueue" ("Q Operations")) -> ("error out"=w448:errorcluster)  [unwired: 11 in, 1 out]
      }
      frame "Exit" {
        n202 = call "Queue Driver.vi"("error in (no error)"=w457, "Queue Operations"=Queue_Operations."Flush" ("Q Operations")) -> ("error out"=w458:errorcluster)  [unwired: 12 in, 1 out]
        n203 = call "Queue Driver.vi"("error in (no error)"=w458, "Queue Operations"=Queue_Operations."Release" ("Q Operations")) -> ("error out"=w459:errorcluster)  [unwired: 12 in, 1 out]
      }
    }
  }
  n204 = invoke class="VI" method="FP.Close"(error in=w6) -> (error out=→"error out":errorcluster)  [unwired: 2 in, 2 out]
